vi "Write Init.vi"(8 "error in (no error)":errorcluster, 10 "Init":bool, 11 "Thorlabs_PM100D in":refnum<class "Thorlabs_PM100D.lvclass">) -> (0 "error out":errorcluster, 3 "Thorlabs_PM100D out":refnum<class "Thorlabs_PM100D.lvclass">)   [LabVIEW 2020, in "Thorlabs_PM100D.lvclass"]
uses:
  <instrlib>/Classes/Powermeter/Thorlabs_PM100D/Thorlabs_PM100D.lvclass
  <instrlib>/Classes/Powermeter/Thorlabs_PM100D/Thorlabs_PM100D.lvclass/Thorlabs_PM100D.ctl
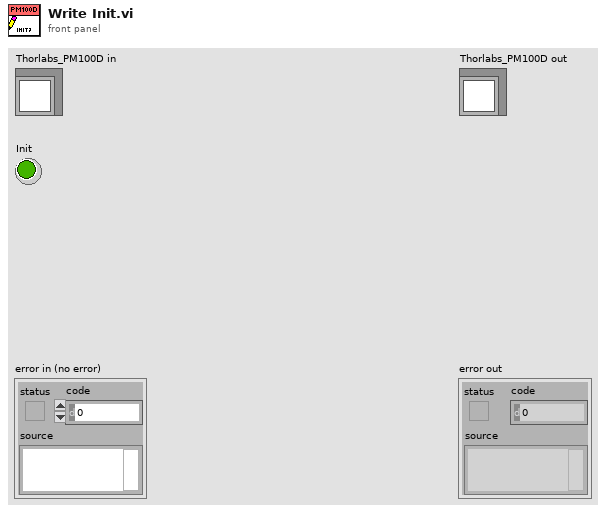
[diagram p1: front panel]
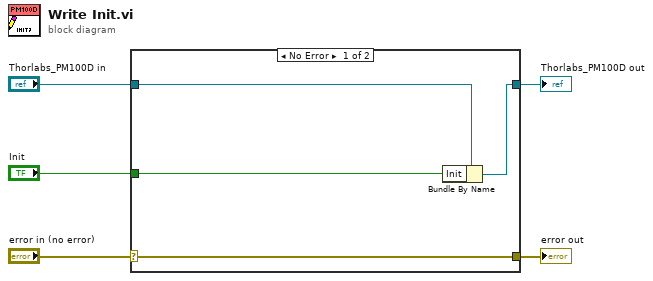
[diagram p0: block diagram]
diagram:
  n1 = case shown="No Error" "error in (no error)" {
    selector: "error in (no error)" -> [w9 w10]
    tunnel: [w9 w10] -> w4
    tunnel: [w7 w11] -> w2
    tunnel: "Thorlabs_PM100D in" -> [w8 w11]
    tunnel: "Init" -> [w6 _]
    frame No Error {
      n2 = Bundle By Name(cluster=w8, "Init"=w6) -> (w7:refnum<class "Thorlabs_PM100D.lvclass">)
    }
    frame Error {
    }
  }
  "error out" <- w4
  "Thorlabs_PM100D out" <- w2
